vi "Overlay Feature Points.vi"(6 "Color":u32(colorbox)=16711680, 7 "Group":string, 8 "error in":errorcluster, 10 "Feature Points":cluster{"X":sgl, "Y":sgl}[](array[cluster]), 11 "Image":T1) -> (0 "error out":errorcluster, 3 "Image Out":T1)   [LabVIEW 2015]
doc: "Overlay targets at the location of the feature points in the specified colors."
uses:
  <vilib>/vision/Image Controls.llb/IMAQ Image.ctl
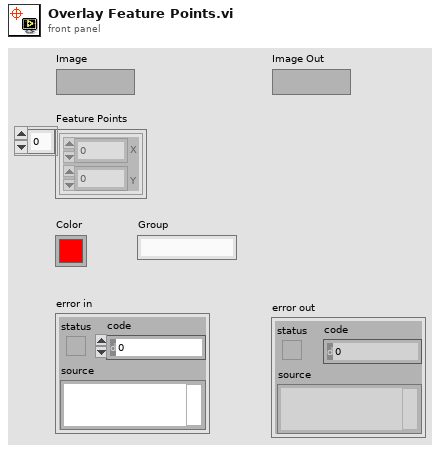
[diagram p1: front panel]
types:
  T1 = typedef "IMAQ Image.ctl" = refnum<image>
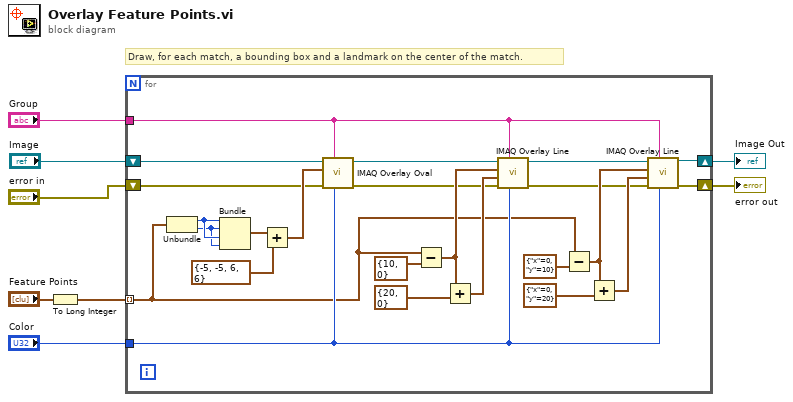
[diagram p0: block diagram]
diagram:
  # "Draw, for each match, a bounding box and a landmark on the center of the match."
  n1 = To Long Integer(number="Feature Points") -> (32bit integer=w5:cluster{"X":i32, "Y":i32}[])
  n2 = for {
    shift-right: [w30] -> w7
    shift-left: "Image" -> [w32]
    tunnel: w5 -> [w9] mode=indexing
    tunnel: "Color" -> [w31]
    tunnel: "Group" -> [w10]
    shift-right: [w11] -> w1
    shift-left: "error in" -> [w14]
    n3 = Unbundle(w9) -> ("X"=w19:i32, "Y"=w18:i32)
    n4 = Bundle("X"=w19, "Y"=w18, "X"=w19, "Y"=w18) -> (w17:cluster{"X":i32, "Y":i32, "X":i32, "Y":i32})  [unwired: 1 in]
    n5 = Add(x=w17, y=cluster{"y":i32, "x":i32, "y":i32, "x":i32} {"y"=-5, "x"=-5, "y"=6, "x"=6}) -> (x+y=w15:cluster{i32, i32, i32, i32})
    n6 = call "IMAQ Overlay Oval"("Color"=w31, "Group"=w10, "error in (no error)"=w14, "Bounding Rectangle"=w15, "Image"=w32) -> ("error out"=w13:errorcluster, "Image Out"=w20:T1)  [unwired: 5 in]
    n7 = Subtract(x=w9, y=cluster{"x":i32, "y":i32} {"x"=10, "y"=0}) -> (x-y=w28:cluster{i32, i32})
    n8 = Add(x=w28, y=cluster{"x":i32, "y":i32} {"x"=20, "y"=0}) -> (x+y=w26:cluster{i32, i32})
    n9 = call "IMAQ Overlay Line"("Color"=w31, "Group"=w10, "error in (no error)"=w13, "End Point"=w26, "Start Point"=w28, "Image"=w20) -> ("error out"=w12:errorcluster, "Image Out"=w21:T1)  [unwired: 4 in]
    n10 = Subtract(x=w9, y=cluster{"x":i32, "y":i32} {"x"=0, "y"=10}) -> (x-y=w24:cluster{i32, i32})
    n11 = Add(x=w24, y=cluster{"x":i32, "y":i32} {"x"=0, "y"=20}) -> (x+y=w25:cluster{i32, i32})
    n12 = call "IMAQ Overlay Line"("Color"=w31, "Group"=w10, "error in (no error)"=w12, "End Point"=w25, "Start Point"=w24, "Image"=w21) -> ("error out"=w11:errorcluster, "Image Out"=w30:T1)  [unwired: 4 in]
  }
  "Image Out" <- w7
  "error out" <- w1
